vi "recallMovesOnRobot.vi"(8 "error in (no error)":errorcluster) -> (3 "Array":T1[](array[typedef]))   [LabVIEW 2017]
uses:
  Auton Control.ctl
panel:
  out "error IO":errorcluster
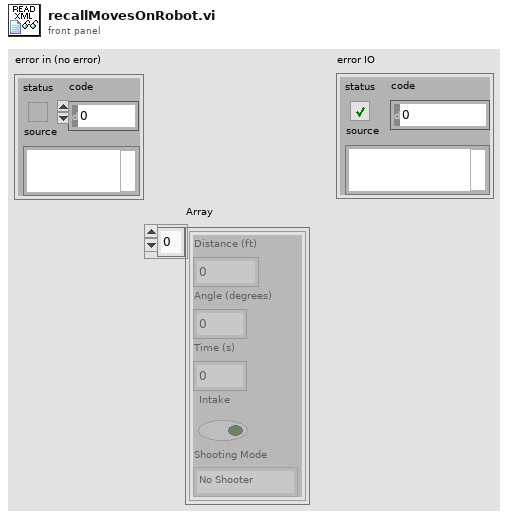
[diagram p1: front panel]
types:
  T1 = typedef "Auton Control.ctl" = cluster{"Distance (ft)":dbl, "Angle (degrees)":dbl, "Time (s)":dbl, "Intake":bool, "Shooting Mode":enum16{"No Shooter", "Low Shooter", "High Shooter"}}
  T2 = enum16{"open", "replace", "create", "open or create", "replace or create", "replace or create with confirmation"}
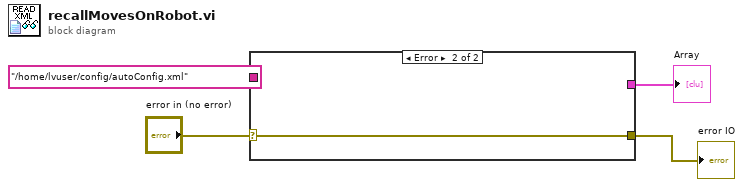
[diagram p0: block diagram]
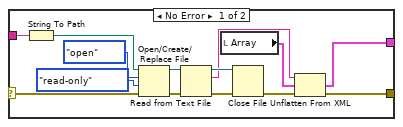
[diagram p2: hidden frame]
diagram:
  n1 = case shown="Error" "error in (no error)" {
    selector: "error in (no error)" -> [w16 w19]
    tunnel: "/home/lvuser/config/autoConfig.xml" -> [w18 _]
    tunnel: [w6 w19] -> w2
    tunnel: [w5 _] -> w1
    frame No Error {
      n2 = String To Path(string=w18) -> (path=w17:path)
      n3 = Open/Create/Replace File(file path (use dialog)=w17, error in=w16, operation (0:open)=T2."open", access (0:read/write)=enum16{"read/write", "read-only", "write-only"}."read-only") -> (refnum out=w13:refnum<file>, error out=w11:errorcluster)  [unwired: 2 in, 1 out]
      n4 = Read from Text File(file (use dialog)=w13, error in=w11) -> (refnum out=w12:refnum<file>, text=w9:string, error out=w10:errorcluster)  [unwired: 2 in, 1 out]
      n5 = local read "Array"() -> (w8:T1[])
      n6 = Close File(refnum=w12, error in=w10) -> (error out=w7:errorcluster)  [unwired: 1 out]
      n7 = Unflatten From XML(xml string=w9, type=w8, error in (no error)=w7) -> (value=w5:T1[], error out=w6:errorcluster)
    }
    frame Error {
    }
  }
  "Array" <- w1
  "error IO" <- w2
